vi "Test wrapper.vi"() -> ()   [LabVIEW 2009]
uses:
  <vilib>/Analysis/2dsp.llb/2D Complex FFT.vi
  <vilib>/Analysis/NI_AALPro.lvlib
panel:
  in  "Intensity":sgl[](array[numeric])=[1.0, 1.0, 1.0]
  in  "Polynomial Coefficients":sgl[](array[numeric])=[128.0, 0.0, 0.0, 40.0, 0.0, 0.0, 0.0, 0.0, 0.0, 0.0, 0.0, 0.0, 0.0, 0.0, 0.0, 0.0, 0.0, 0.0, 0.0, 0.0, 0.0, 0.0, 0.0, 0.0, 0.0, 0.0, 0.0, 0.0, 0.0, 0.0, 0.0, 0.0, 0.0, 0.0, 0.0, 0.0, 0.0, 0.0, 0.0, 0.0, 0.0, 0.0, 0.0, 0.0, 0.0, 0.0, 0.0, 0.0, 0.0, 0.0, 0.0, 0.0, 0.0, 0.0, 0.0, 0.0, 0.0, 0.0, 0.0, 0.0, 0.0, 0.0, 0.0, 0.0, 0.0, 0.0, 0.0, 0.0, 0.0, 0.0, 0.0, 0.0, 0.0, 0.0, 0.0, 0.0, 0.0, 0.0, 0.0, 0.0, 0.0, 0.0, 0.0, 0.0, 0.0, 0.0, 0.0, 0.0, 0.0, 0.0, 0.0, 0.0, 0.0, 0.0, 0.0, 0.0, 0.0, 0.0, 0.0, 0.0, 0.0, 0.0, 0.0, 0.0, 0.0, 0.0, 0.0, 0.0, 0.0, 0.0, 0.0, 0.0, 0.0, 0.0, 0.0, 0.0, 0.0, 0.0, 0.0, 0.0]
  in  "alpha RPC":sgl=1.0
  in  "Polynomial Order":i32=3 min=3 max=7 step=1
  in  "Use polynomial LUT":bool=TRUE
  out "error out":errorcluster
  in  "Aberration Correction On":bool
  in  "Aberration Correction":sgl[](array[numeric])=array[262144 elements]
  in  "TrueFrame":i32=3
  in  "Number of \ntime to execute":i32=1
  out "Average \nexecution time":dbl=nan
  in  "GO":bool
  in  "stop program":bool
  out "Amplitudes/weights":sgl[][](graph)=[[1.0001239, 1.0001477, 1.0001446, 1.0001416, 1.0001386, 1.0001358, 1.0001332, 1.0001305, 1.0001283, 1.0001258], [0.99984175, 0.99979293, 0.9997994, 0.99980545, 0.9998114, 0.9998169, 0.9998223, 0.99982744, 0.9998326, 0.9998372], [1.0000381, 1.0000628, 1.0000595, 1.0000563, 1.0000532, 1.0000505, 1.0000477, 1.0000453, 1.0000426, 1.0000404]]
  out "Calculated image plane":dbl[][](graph)
  out "Generated Hologram":u8[][](graph)
  in  "method":i32(ring)=1 items=["Lenses and Gratings (3D)", "Gerchberg-Saxton (3D)", "Gerchberg-Saxton FFT (2D)"]
  in  "z":sgl[](array[numeric])=[0.0, 0.0, 0.0]
  in  "y":sgl[](array[numeric])=[4.0, 5.0, -4.0]
  in  "x":sgl[](array[numeric])=[4.0, -4.0, 4.0]
  in  "N_iterations":i32=10
  in  "SLM enabled":bool
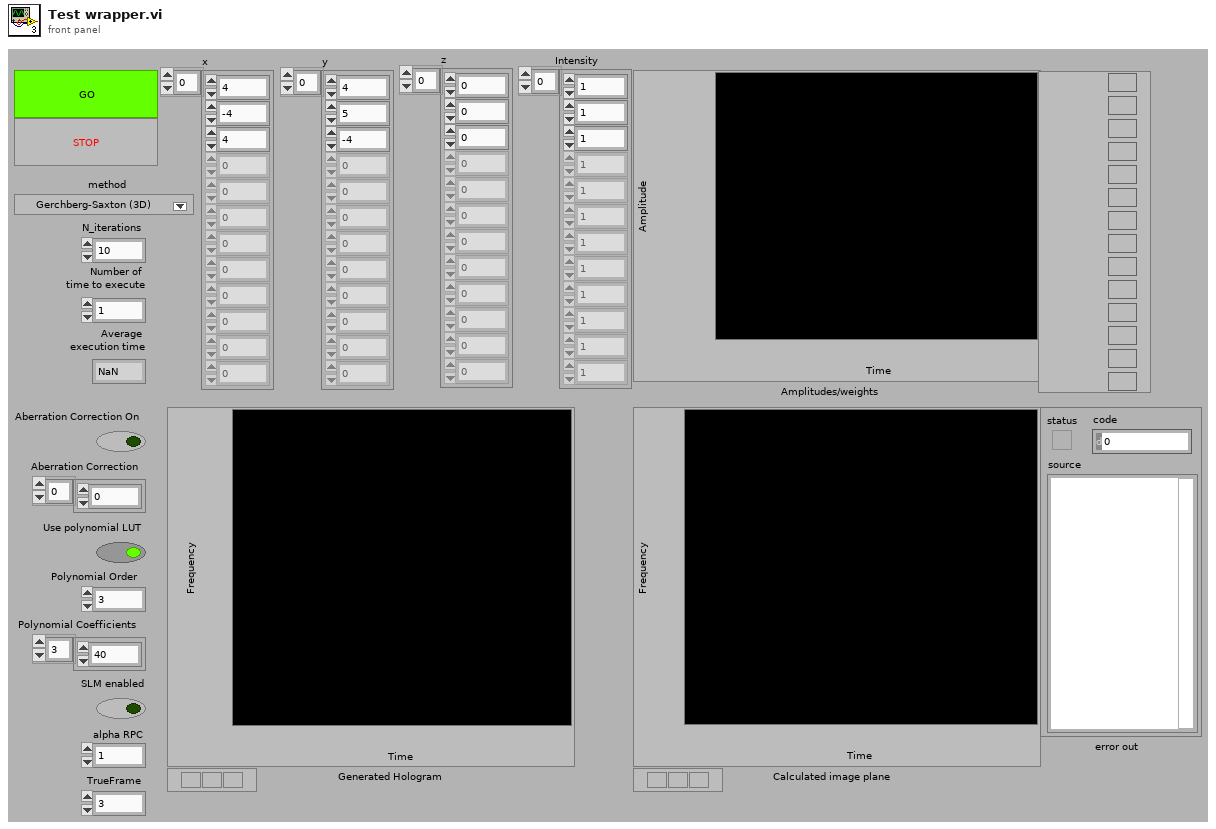
[diagram p1: front panel]
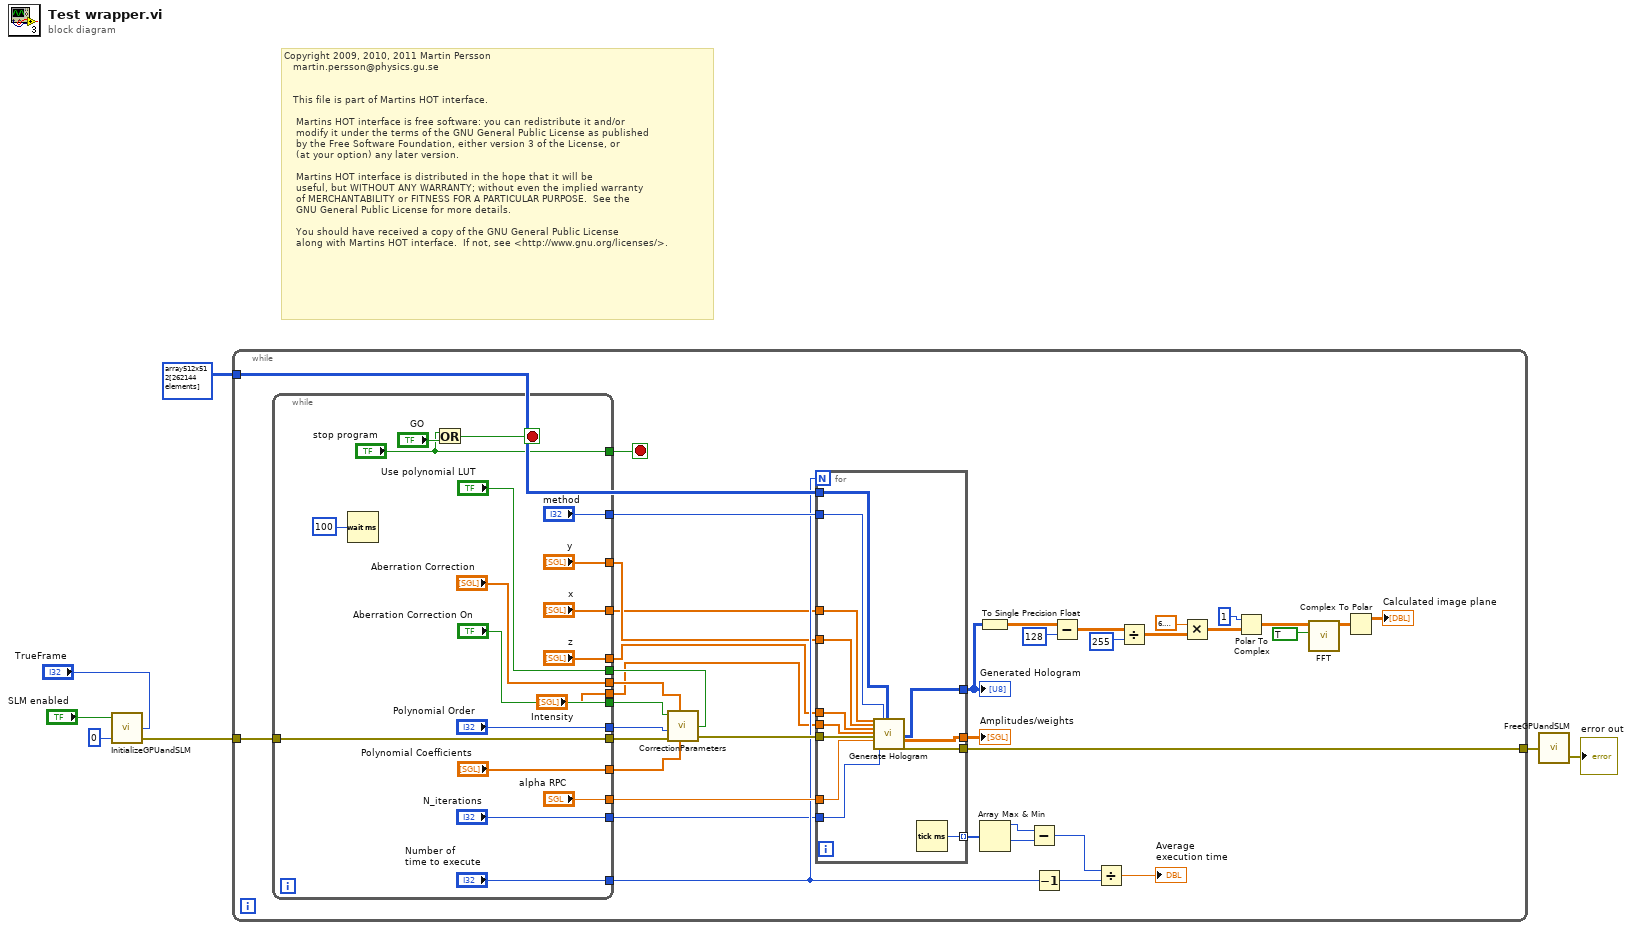
[diagram p0: block diagram]
diagram:
  # "Copyright 2009, 2010, 2011 Martin Persson \n   martin.persson@physics.gu.se\n\n\n   This file is part of Martins HOT interface.\n\n    Martins HOT interface is free software: you can redistribute it and/or \n    modify it under the terms of the GNU General Public License as published \n    by the Free Software Foundation, either version 3 of the License, or\n    (at your option) any later version.\n\n    Martins HOT interface is distributed in the hope that it will be \n    useful, but WITHOUT ANY WARRANTY; without even the implied warranty\n    of MERCHANTABILITY or FITNESS FOR A PARTICULAR PURPOSE.  See the\n    GNU General Public License for more details.\n\n    You should have received a copy of the GNU General Public License\n    along with Martins HOT interface.  If not, see <http://www.gnu.org/licenses/>."
  n1 = call "InitializeGPUandSLM.vi"("TrueFrame"="TrueFrame", "deviceId"=0 ("SLM size"), "SLM enabled"="SLM enabled") -> ("CUDA/SLM error"=w1:errorcluster)  [unwired: 1 in, 1 out]
  n2 = while {
    tunnel: w1 -> [w23]
    tunnel: [w44] -> w6
    tunnel: u8[][] array512x512[262144 elements] ("Default") -> [w31]
    stop <- w45 stop-if-true
    n3 = while {
      tunnel: ["stop program"] -> w45
      tunnel: w23 -> [w73]
      tunnel: [w73] -> w22
      tunnel: ["alpha RPC"] -> w20
      tunnel: ["Use polynomial LUT"] -> w19
      tunnel: ["Aberration Correction On"] -> w18
      tunnel: ["method"] -> w17
      tunnel: ["Number of \ntime to execute"] -> w16
      tunnel: ["y"] -> w15
      tunnel: ["z"] -> w14
      tunnel: ["x"] -> w13
      tunnel: ["Polynomial Order"] -> w12
      tunnel: ["Aberration Correction"] -> w11
      tunnel: ["Polynomial Coefficients"] -> w10
      tunnel: ["N_iterations"] -> w9
      tunnel: ["Intensity"] -> w8
      stop <- w75 stop-if-true
      n4 = Wait (ms)(milliseconds to wait=u32 100) -> ()  [unwired: 1 out]
      n5 = Or(x="stop program", y="GO") -> (x .or. y?=w75:bool)
    }
    n6 = call "CorrectionParameters.vi"("Aberration Correction On"=w18, "Aberration Correction"=w11, "Polynomial Order"=w12, "Polynomial Coefficients"=w10, "error in"=w22, "Use polynomial LUT"=w19) -> ("error out"=w24:errorcluster)  [unwired: 1 in, 1 out]
    n7 = for {
      N: w16 -> [_]
      tunnel: w24 -> [w59]
      tunnel: w9 -> [w58]
      tunnel: w15 -> [w57]
      tunnel: w14 -> [w56]
      tunnel: w17 -> [w55]
      tunnel: [w54] -> w46
      tunnel: [w53] -> w44
      tunnel: [w52] -> w32
      tunnel: w31 -> [w51]
      tunnel: w13 -> [w50]
      tunnel: w8 -> [w49]
      tunnel: [w48] -> w30 mode=indexing
      tunnel: w20 -> [w47]
      n8 = call "Generate Hologram.vi"("x"=w50, "y"=w57, "z"=w56, "spot_intensities"=w49, "CUDA/SLM error in"=w59, "alpha RPC"=w47, "N_iterations"=w58, "method"=w55, "CGH in"=w51) -> ("CGH out"=w52:u8[][], "weights"=w54:sgl[][], "CUDA/SLM error out"=w53:errorcluster)  [unwired: 16 in]
      n9 = Tick Count (ms)() -> (millisecond timer value=w48:u32)
    }
    "Generated Hologram" <- w32
    "Amplitudes/weights" <- w46
    n10 = To Single Precision Float(number=w32) -> (single precision float=w39:sgl[][])
    n11 = Array Max & Min(array=w30) -> (max value=w29:u32, min value=w28:u32)  [unwired: 2 out]
    n12 = Subtract(x=w29, y=w28) -> (x-y=w27:u32)
    n13 = Decrement(x=w16) -> (x-1=w21:i32)
    n14 = Subtract(x=w39, y=128) -> (x-y=w38:sgl[][])
    n15 = Divide(x=w27, y=w21) -> (x/y=→"Average \nexecution time":dbl)
    n16 = Divide(x=w38, y=255) -> (x/y=w41:sgl[][])
    n17 = Multiply(x=6.283185307179586, y=w41) -> (x*y=w35:dbl[][])
    n18 = Polar To Complex(1:w35, 2:1) -> (0:w34:cdb[][])
    n19 = call-poly <vilib>:"FFT.vi"("shift?"=TRUE, "X"=w34) -> ("FFT {X}"=w37:cdb[][])  [unwired: 2 in, 7 out]
    n20 = Complex To Polar(r * e^(i*theta)=w37) -> (r=→"Calculated image plane":dbl[][])  [unwired: 1 out]
  }
  n21 = call "FreeGPUandSLM.vi"("error in"=w6) -> ("error out"=→"error out":errorcluster)  [unwired: 1 out]
